vi "Target Test.vi"() -> ()   [LabVIEW 2012]
uses:
  <vilib>/rvi/eio/common/nirviEmuTemplateMethod_errors.vi
  <vilib>/rvi/interface/RandomDataEmulation/nirviRandomDataFPGAFIFO.vi
  <vilib>/rvi/interface/RandomDataEmulation/niFpgaRandomDataHandleErrors.vi
  <vilib>/eio/EIONode/EIONode.xnode
  <vilib>/rvi/DataTransferAndStorage/Container/XNode/niFpgaContainer.xnode
  <vilib>/rvi/interface/RandomDataEmulation/nirviRandomDataFpgaReadWriteTemplate.vi
panel:
  out "FPGA Voltage Indicator":i16
  in  "Host Output Voltage":i16
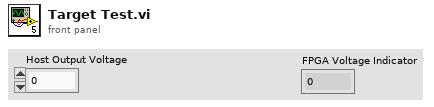
[diagram p1: front panel]
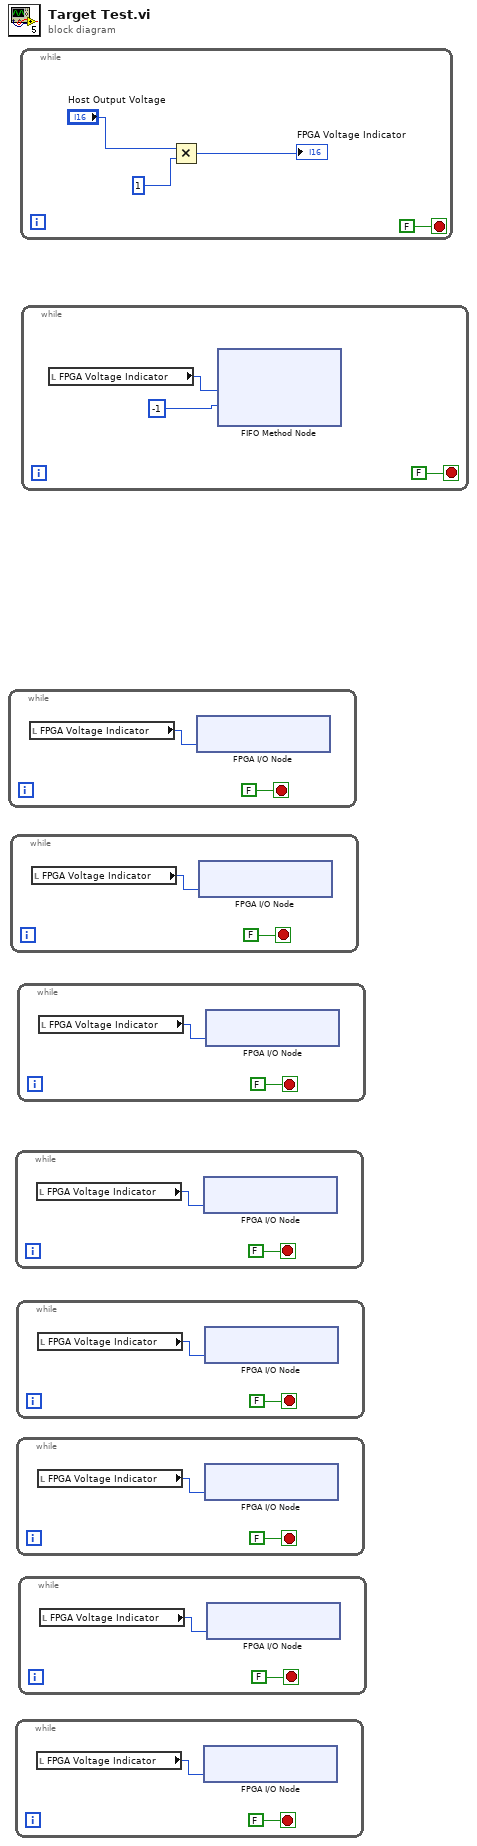
[diagram p0: block diagram]
diagram:
  n1 = while {
    stop <- FALSE stop-if-true
    n2 = local read "FPGA Voltage Indicator"() -> (w1:i16)
    n3 = xnode "FPGA I/O Node"("Connector0/AO0"=w1) -> ()  [unwired: 1 in, 1 out]
  }
  n4 = while {
    stop <- FALSE stop-if-true
    n5 = local read "FPGA Voltage Indicator"() -> (w3:i16)
    n6 = xnode "FPGA I/O Node"("Connector0/AO1"=w3) -> ()  [unwired: 1 in, 1 out]
  }
  n7 = while {
    stop <- FALSE stop-if-true
    n8 = local read "FPGA Voltage Indicator"() -> (w5:i16)
    n9 = xnode "FPGA I/O Node"("Connector0/AO3"=w5) -> ()  [unwired: 1 in, 1 out]
  }
  n10 = while {
    stop <- FALSE stop-if-true
    n11 = local read "FPGA Voltage Indicator"() -> (w7:i16)
    n12 = xnode "FPGA I/O Node"("Connector0/AO7"=w7) -> ()  [unwired: 1 in, 1 out]
  }
  n13 = while {
    stop <- FALSE stop-if-true
    n14 = local read "FPGA Voltage Indicator"() -> (w9:i16)
    n15 = xnode "FPGA I/O Node"("Connector0/AO4"=w9) -> ()  [unwired: 1 in, 1 out]
  }
  n16 = while {
    stop <- FALSE stop-if-true
    n17 = local read "FPGA Voltage Indicator"() -> (w11:i16)
    n18 = xnode "FPGA I/O Node"("Connector0/AO5"=w11) -> ()  [unwired: 1 in, 1 out]
  }
  n19 = while {
    stop <- FALSE stop-if-true
    n20 = local read "FPGA Voltage Indicator"() -> (w13:i16)
    n21 = xnode "FPGA I/O Node"("Connector0/AO2"=w13) -> ()  [unwired: 1 in, 1 out]
  }
  n22 = while {
    stop <- FALSE stop-if-true
    n23 = local read "FPGA Voltage Indicator"() -> (w15:i16)
    n24 = xnode "FPGA I/O Node"("Connector0/AO6"=w15) -> ()  [unwired: 1 in, 1 out]
  }
  n25 = while {
    stop <- FALSE stop-if-true
    n26 = Multiply(x="Host Output Voltage", y=i16 1) -> (x*y=→"FPGA Voltage Indicator":i16)
  }
  n27 = while {
    stop <- FALSE stop-if-true
    n28 = local read "FPGA Voltage Indicator"() -> (w21:i16)
    n29 = xnode ("FIFO Method Node")("Element"=w21, "Timeout"=i16 -1) -> ()  [unwired: 1 in, 2 out]
  }
